vi "TestApplication.vi"() -> ()   [LabVIEW 2016]
uses:
  SEDSpectrometer/FiberSpectrograph.lvclass
  <vilib>/express/express arith-compare/Formula/XNode/ExpressFormulaBlockNode.xnode
panel:
  in  "NrOfAVG":u32=1 caption="Number of averages"
  in  "IntDelay":dbl=-20.0 caption="Integration delay [ns]" min=-20.0 format="%#.0f"
  in  "IntTime":sgl=32.0 caption="Integration time [ms]" format="%.2f"
  out "TecControlType.Setpoint":sgl
  in  "Get Temp Setpoint":bool
  in  "Get Temperature":bool caption="Start Measurement"
  out "Current Temperature":sgl=-6.1035157e-06 format="%_2f"
  in  "Set Parameters":bool caption="Start Measurement"
  in  "Temperature Setpoint":sgl=1.0 format="%_3f"
  out "XY Graph":cluster{"Y":dbl[], "Y":dbl[]}[](graph)
  in  "Exit":bool
  out "Status":string
  in  "StopMeasurement":bool
  in  "StartMeasurement":bool caption="Start Measurement"
  in  "NrOfScans":i16=-1 caption="Nr Of Scans"
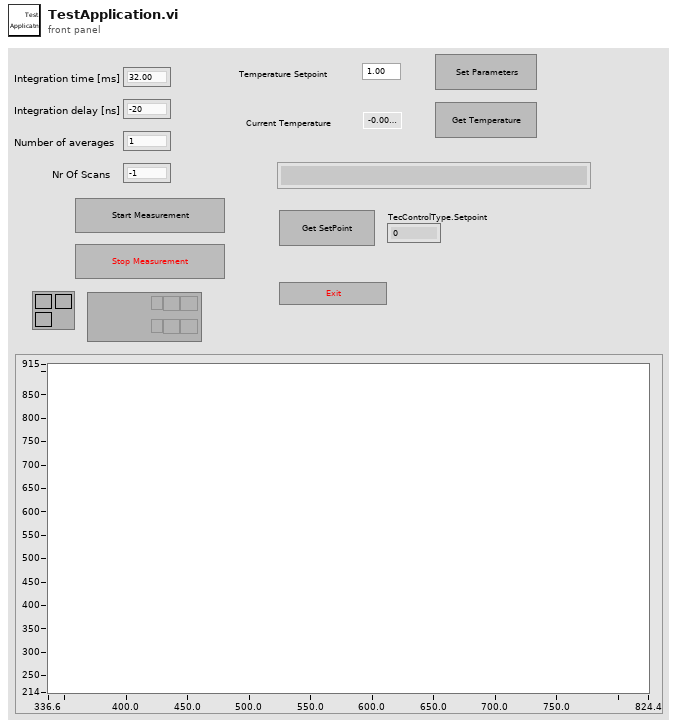
[diagram p1: front panel]
types:
  T1 = cluster{"StartPixel":u16, "StopPixel":u16, "IntegrationTime":sgl, "IntegrationDelay":u32, "NrAverages":u32, "DarkCorrectionType":cluster{"Enable CorDynDark":u8, "ForgetPercentage":u8}, "SmoothingType":cluster{"SmoothPix":u16, "SmoothModel":u8}, "SatDetection":u8, "TriggerType":cluster{"Trigger Mode":u8, "Trigger Source":u8, "Trigger SourceType":u8}, "ControlSettingsType":cluster{"StrobeControl":u16, "LaserDelay":u32, "LaserWidth":u32, "LaserWaveLength":sgl, "StoreToRam":u16}}
  T2 = cluster{"Len":u16, "ConfigVersion":u16, "UserFriendlyId":u8[], "DetectorType":cluster{"SensorType":u8, "NrPixels":u16, "Fit":sgl[], "NLEnable":u8, "NLCorrect":dbl[], "LowNLCounts":dbl, "HighNLCounts":dbl, "Gain":sgl[], "Reserved":sgl, "Offset":sgl[], "Extern Offset":sgl, "DefectivePixels":u16[]}, "IrradianceType":cluster{"SpectrumCalibrationType":cluster{"SmoothingType":cluster{"m_SmoothPix":u16, "SmoothModel":u8}, "CalInttime":sgl, "CalibConvers":sgl[]}, "CalibrationType":u8, "FiberDiameter":i32}, "SpectrumCalibrationType":cluster{"SmoothingType":cluster{"m_SmoothPix":u16, "SmoothModel":u8}, "CalInttime":sgl, "CalibConvers":sgl[]}, "SpectrumCorrectionType":sgl[], "StandAloneType":cluster{"StandAloneType":u8, "MeasConfigType":cluster{"StartPixel":u16, "StopPixel":u16, "IntegrationTime":sgl, "IntegrationDelay":u32, "NrAverages":u32, "DarkCorrectionType":cluster{"Enable CorDynDark":u8, "ForgetPercentage":u8}, "SmoothingType":cluster{"SmoothPix":u16, "SmoothModel":u8}, "SatDetection":u8, "TriggerType":cluster{"Trigger Mode":u8, "Trigger Source":u8, "Trigger SourceType":u8}, "ControlSettingsType":cluster{"StrobeControl":u16, "LaserDelay":u32, "LaserWidth":u32, "LaserWaveLength":sgl, "StoreToRam":u16}}, "Nmsr":i16}, "DynamicStorageType":cluster{"Nmsr":i32, "Reserved":u8[]}, "TempSensorType":sgl[], "TecControlType":cluster{"Enable":u8, "Setpoint":sgl, "Fit[NR_DAC_POL_COEF]":sgl[]}, "ProcessControlType":cluster{"AnalogLow":sgl[], "AnalogHigh":sgl[], "DigitalLow":sgl[], "DigitalHigh":sgl[]}, "EthernetSettingsType":cluster{"IpAddr":u32, "NetMask":u32, "Gateway":u32, "DhcpEnabled":u8, "TcpPort":u16, "LinkStatus":u8}, "Reserved":u8[]}
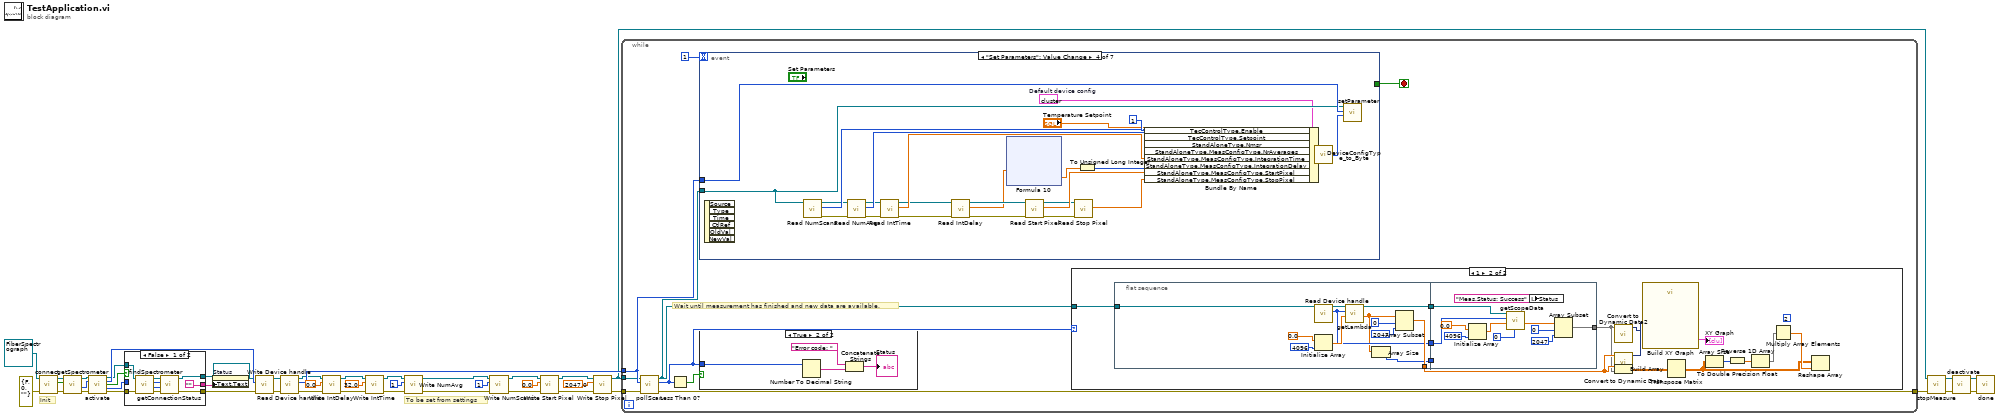
[diagram p0: block diagram]
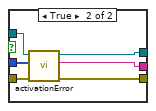
[diagram p2: hidden frame]
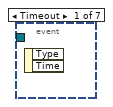
[diagram p5: hidden frame]
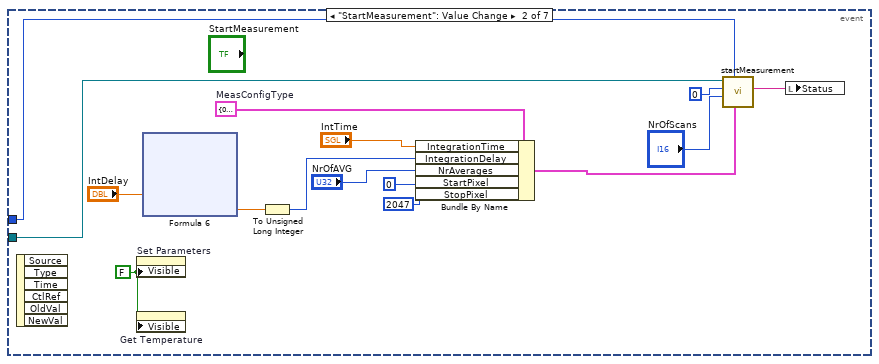
[diagram p6: hidden frame]
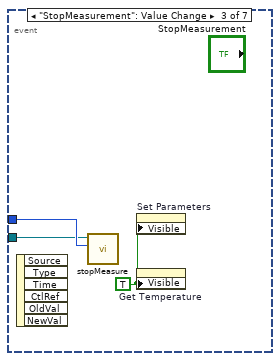
[diagram p7: hidden frame]
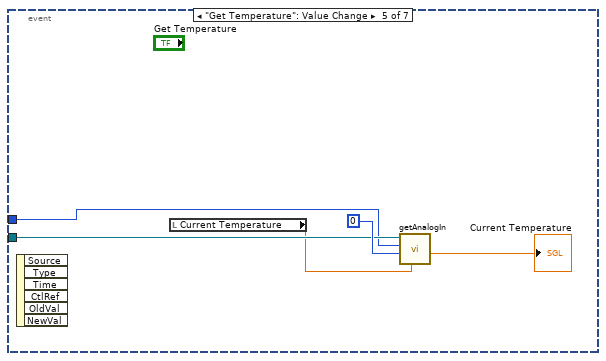
[diagram p8: hidden frame]
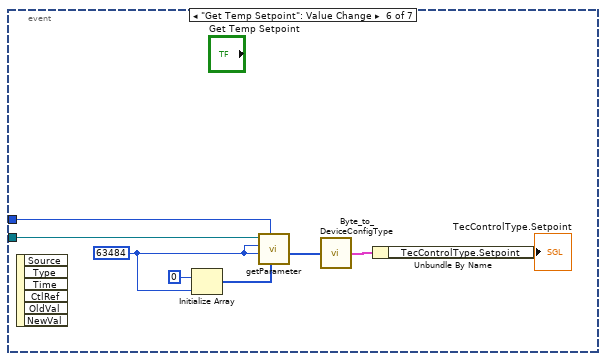
[diagram p9: hidden frame]
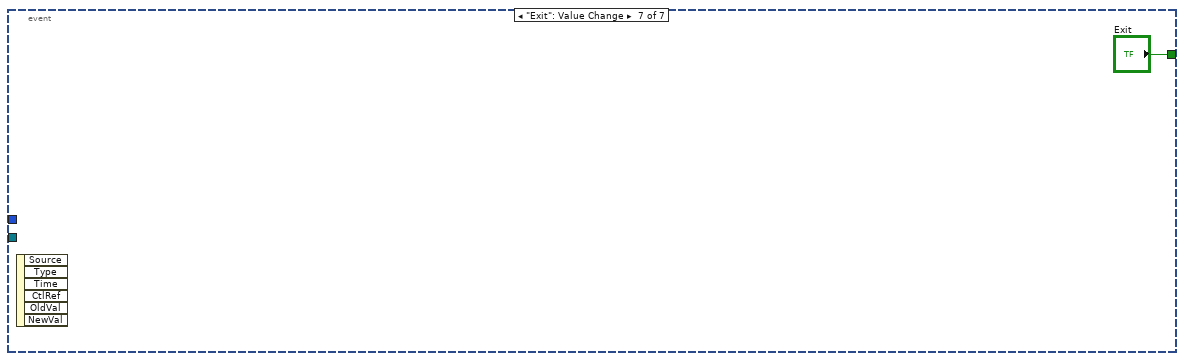
[diagram p10: hidden frame]
diagram:
  # "To be set from settings"
  # "Init"
  n1 = call "connect.vi"("error in (no error)"=errorcluster {"status"=FALSE, "code"=0, "source"=""}, "SEDSpectrometer in"=refnum<class "FiberSpectrograph.lvclass"> refnum) -> ("error out"=w41:errorcluster, "Connected"=w22:bool, "SEDSpectrometer out"=w42:refnum<class "FiberSpectrograph.lvclass">)  [unwired: 7 in]
  n2 = call "getSpectrometer.vi"("error in (no error)"=w41, "Boolean"=w22, "SEDSpectrometer in"=w42) -> ("error out"=w37:errorcluster, "AviableSpec"=w40:u8[], "SEDSpectrometer out"=w36:refnum<class "FiberSpectrograph.lvclass">)  [unwired: 6 in]
  n3 = call "activate.vi"("SEDSpectrometer in"=w36, "DeviceId"=w40, "error in (no error)"=w37) -> ("SEDSpectrometer out"=w30:refnum<class "FiberSpectrograph.lvclass">, "Device handle"=w31:i32, "Activation Error"=w26:bool, "DeviceId"=w27:u8[], "error out"=w29:errorcluster)  [unwired: 8 in]
  n4 = case shown="False" w26 {
    tunnel: w30 -> [w52 w59]
    tunnel: w29 -> [w51 w58]
    tunnel: [w47 w57] -> w24
    tunnel: ["" ("Status") w56] -> w28
    tunnel: w27 -> [_ w55]
    tunnel: [w46 w54] -> w25
    frame False {
      n5 = call "findSpectrometer.vi"("error in (no error)"=w51, "SEDSpectrometer in"=w52) -> ("error out"=w48:errorcluster, "NumOfDevices"=w49:i32, "AviableSpec"=w50:u8[], "SEDSpectrometer out"=w53:refnum<class "FiberSpectrograph.lvclass">)  [unwired: 6 in]
      n6 = call "getConnectionStatus.vi"("SEDSpectrometer in"=w53, "AvailableSpectrometer"=w50, "NumOfDevices"=w49, "error in (no error)"=w48) -> ("SEDSpectrometer out"=w46:refnum<class "FiberSpectrograph.lvclass">, "error out"=w47:errorcluster)  [unwired: 4 in, 1 out]
    }
    frame True {
      n7 = call "activationError.vi"("error in (no error)"=w58, "DeviceId"=w55, "SEDSpectrometer in"=w59) -> ("error out"=w57:errorcluster, "Status"=w56:string, "SEDSpectrometer out"=w54:refnum<class "FiberSpectrograph.lvclass">)  [unwired: 6 in]
    }
  }
  n8 = property on="Status" class="Str"("Text.Text"=w28) -> ()  [unwired: 2 in, 2 out]
  n9 = call-dynamic "Write Device handle.vi"("error in (no error)"=w24, "Device handle"=w31, "SEDSpectrometer in"=w25) -> ("error out"=w35:errorcluster, "SEDSpectrometer out"=w32:refnum<class "FiberSpectrograph.lvclass">)  [unwired: 7 in]
  n10 = call-dynamic "Read Device handle.vi"("error in (no error)"=w35, "SEDSpectrometer in"=w32) -> ("error out"=w7:errorcluster, "Device handle"=w21:i32, "SEDSpectrometer out"=w2:refnum<class "FiberSpectrograph.lvclass">)  [unwired: 7 in]
  n11 = call-dynamic "Write IntDelay.vi"("error in (no error)"=w7, "IntDelay"=0.0, "SEDSpectrometer in"=w2) -> ("error out"=w15:errorcluster, "SEDSpectrometer out"=w20:refnum<class "FiberSpectrograph.lvclass">)  [unwired: 7 in]
  n12 = call-dynamic "Write IntTime.vi"("error in (no error)"=w15, "IntTime"=sgl 32.0, "SEDSpectrometer in"=w20) -> ("error out"=w14:errorcluster, "SEDSpectrometer out"=w19:refnum<class "FiberSpectrograph.lvclass">)  [unwired: 7 in]
  n13 = call-dynamic "Write NumAvg.vi"("error in (no error)"=w14, "NumAvg"=u32 1, "SEDSpectrometer in"=w19) -> ("error out"=w13:errorcluster, "SEDSpectrometer out"=w18:refnum<class "FiberSpectrograph.lvclass">)  [unwired: 7 in]
  n14 = call-dynamic "Write NumScans.vi"("error in (no error)"=w13, "NumScans"=i16 1, "SEDSpectrometer in"=w18) -> ("error out"=w12:errorcluster, "SEDSpectrometer out"=w17:refnum<class "FiberSpectrograph.lvclass">)  [unwired: 7 in]
  n15 = call-dynamic "Write Start Pixel.vi"("error in (no error)"=w12, "Start Pixel"=0.0, "SEDSpectrometer in"=w17) -> ("error out"=w11:errorcluster, "SEDSpectrometer out"=w16:refnum<class "FiberSpectrograph.lvclass">)  [unwired: 7 in]
  n16 = call-dynamic "Write Stop Pixel .vi"("error in (no error)"=w11, "Stop Pixel"=2047.0, "SEDSpectrometer in"=w16) -> ("error out"=w6:errorcluster, "SEDSpectrometer out"=w1:refnum<class "FiberSpectrograph.lvclass">)  [unwired: 7 in]
  n17 = while {
    tunnel: w21 -> [w61]
    tunnel: w6 -> [w65]
    tunnel: [w64] -> w23
    tunnel: w1 -> [w60]
    stop <- w66 stop-if-true
    # "Wait until measurement has finished and new data are available."
    n18 = call "pollScan.vi"("error in (no error)"=w65, "Device"=w61, "SEDSpectrometer in"=w60) -> ("error out"=w64:errorcluster, "Output Value"=w62:i32, "SEDSpectrometer out"=w63:refnum<class "FiberSpectrograph.lvclass">)  [unwired: 6 in]
    n19 = Less Than 0?(x=w62) -> (x < 0?=w67:bool)
    n20 = event shown="[3] \"Set Parameters\": Value Change" {
      selector: _ -> [_ _ _ _ _ _ _]
      dyn-events: _ -> [_ _ _ _ _ _ _]
      timeout: 1 -> [_ _ _ _ _ _ _]
      tunnel: [_ _ _ _ _ _ "Exit"] -> w66
      tunnel: w61 -> [_ w125 w136 w144 w172 w178 _]
      tunnel: w63 -> [_ w121 w135 w143 w173 w175 _]
      event Timeout {
        n21 = event-data() -> ()  [unwired: 1 in, 2 out]
      }
      event "StartMeasurement": Value Change {
        w119 = T1 {"StartPixel"=0, "StopPixel"=0, "IntegrationTime"=0.0, "IntegrationDelay"=0, "NrAverages"=0, "DarkCorrectionType"={"Enable CorDynDark"=0, "ForgetPercentage"=0}, "SmoothingType"={"SmoothPix"=0, "SmoothModel"=0}, "SatDetection"=0, "TriggerType"={"Trigger Mode"=0, "Trigger Source"=0, "Trigger SourceType"=0}, "ControlSettingsType"={"StrobeControl"=0, "LaserDelay"=0, "LaserWidth"=0, "LaserWaveLength"=0.0, "StoreToRam"=0}}  # MeasConfigType
        w120 = FALSE ("Visible")
        n22 = event-data() -> ()  [unwired: 1 in, 6 out]
        n23 = property on="Set Parameters" class="Bool"("Visible"=w120) -> ()  [unwired: 2 in, 2 out]
        n24 = property on="Get Temperature" class="Bool"("Visible"=w120) -> ()  [unwired: 2 in, 2 out]
        n25 = xnode "Formula 6"("X1"="IntDelay") -> ("Result"=w116:dbl)  [unwired: 1 in, 1 out]
        n26 = To Unsigned Long Integer(number=w116) -> (unsigned 32bit integer=w115:u32)
        n27 = Bundle By Name(cluster=w119, "IntegrationTime"="IntTime", "IntegrationDelay"=w115, "NrAverages"="NrOfAVG", "StartPixel"=u16 0, "StopPixel"=2047 ("length")) -> (w111:T1)
        n28 = call "startMeasurement.vi"("MeasConfigType"=w111, "Device Handle"=w125, "NumOfScans"="NrOfScans", "a_hWnd"=0, "SEDSpectrometer in"=w121) -> ("Status"=w122:string)  [unwired: 3 in, 3 out]
        n29 = local write "Status"(w122) -> ()
      }
      event "StopMeasurement": Value Change {
        w134 = TRUE ("Visible")
        n30 = event-data() -> ()  [unwired: 1 in, 6 out]
        n31 = call "stopMeasure.vi"("Device"=w136, "SEDSpectrometer in"=w135) -> ()  [unwired: 7 in, 3 out]
        n32 = property on="Set Parameters" class="Bool"("Visible"=w134) -> ()  [unwired: 2 in, 2 out]
        n33 = property on="Get Temperature" class="Bool"("Visible"=w134) -> ()  [unwired: 2 in, 2 out]
      }
      event "Set Parameters": Value Change {
        w140 = T2 {"Len"=63484, "ConfigVersion"=3, "UserFriendlyId"=[49, 54, 48, 54, 49, 57, 50, 85, 49, 0, 48, 0, 28, 0, 0, 0, 42, 2, 0, 0, 160, 188, 0, 0, 0, 28, 0, 6, 132, 159, 116, 3, 172, 0, 116, 6, 140, 0, 0, 0, 0, 0, 0, 255, 8, 0, 67, 176, 96, 0, 252, 0, 0, 0, 254, 175, 38, 0, 0, 0, 184, 239, 0, 0], "DetectorType"={"SensorType"=11, "NrPixels"=2048, "Fit"=[314.9799, 0.2943957, -9.917037e-06, -1.0080056e-09, 0.0], "NLEnable"=0, "NLCorrect"=[0.0, 0.0, 0.0, 0.0, 0.0, 0.0, 0.0, 0.0], "LowNLCounts"=0.0, "HighNLCounts"=0.0, "Gain"=[1.277, 1.0], "Reserved"=0.0, "Offset"=[-0.01, 0.0], "Extern Offset"=0.0, "DefectivePixels"=[4095, 4095, 4095, 4095, 4095, 4095, 4095, 4095, 4095, 4095, 4095, 4095, 4095, 4095, 4095, 4095, 4095, 4095, 4095, 4095, 4095, 4095, 4095, 4095, 4095, 4095, 4095, 4095, 4095, 4095]}, "IrradianceType"={"SpectrumCalibrationType"={"SmoothingType"={"m_SmoothPix"=0, "SmoothModel"=0}, "CalInttime"=0.0, "CalibConvers"=array[4096 elements]}, "CalibrationType"=0, "FiberDiameter"=0}, "SpectrumCalibrationType"={"SmoothingType"={"m_SmoothPix"=0, "SmoothModel"=0}, "CalInttime"=0.0, "CalibConvers"=array[4096 elements]}, "SpectrumCorrectionType"=array[4096 elements], "StandAloneType"={"StandAloneType"=0, "MeasConfigType"={"StartPixel"=0, "StopPixel"=2047, "IntegrationTime"=32.0, "IntegrationDelay"=0, "NrAverages"=1, "DarkCorrectionType"={"Enable CorDynDark"=1, "ForgetPercentage"=100}, "SmoothingType"={"SmoothPix"=0, "SmoothModel"=0}, "SatDetection"=1, "TriggerType"={"Trigger Mode"=0, "Trigger Source"=0, "Trigger SourceType"=0}, "ControlSettingsType"={"StrobeControl"=0, "LaserDelay"=0, "LaserWidth"=0, "LaserWaveLength"=0.0, "StoreToRam"=0}}, "Nmsr"=-1}, "DynamicStorageType"={"Nmsr"=0, "Reserved"=[0, 0, 0, 0, 0, 0, 0, 0]}, "TempSensorType"=[118.68976, -70.361015, 21.019672, -3.6442714, 0.1992981, 0.0, 0.0, 0.0, 0.0, 0.0, 51.4, -16.38, 0.0, 0.0, 0.0], "TecControlType"={"Enable"=1, "Setpoint"=1.0, "Fit[NR_DAC_POL_COEF]"=[0.0, 0.0]}, "ProcessControlType"={"AnalogLow"=[0.0, 0.0], "AnalogHigh"=[0.0, 0.0], "DigitalLow"=[0.0, 0.0, 0.0, 0.0, 0.0, 0.0, 0.0, 0.0, 0.0, 0.0], "DigitalHigh"=[0.0, 0.0, 0.0, 0.0, 0.0, 0.0, 0.0, 0.0, 0.0, 0.0]}, "EthernetSettingsType"={"IpAddr"=0, "NetMask"=0, "Gateway"=0, "DhcpEnabled"=0, "TcpPort"=0, "LinkStatus"=0}, "Reserved"=array[13815 elements]}  # Default device config
        n34 = event-data() -> ()  [unwired: 1 in, 6 out]
        n35 = call-dynamic "Read NumScans.vi"("SEDSpectrometer in"=w143) -> ("error out"=w158:errorcluster, "NumScans"=w159:i16, "SEDSpectrometer out"=w157:refnum<class "FiberSpectrograph.lvclass">)  [unwired: 8 in]
        n36 = call-dynamic "Read NumAvg.vi"("error in (no error)"=w158, "SEDSpectrometer in"=w157) -> ("error out"=w155:errorcluster, "NumAvg"=w156:u32, "SEDSpectrometer out"=w154:refnum<class "FiberSpectrograph.lvclass">)  [unwired: 7 in]
        n37 = call-dynamic "Read IntTime.vi"("error in (no error)"=w155, "SEDSpectrometer in"=w154) -> ("error out"=w152:errorcluster, "IntTime"=w153:sgl, "SEDSpectrometer out"=w151:refnum<class "FiberSpectrograph.lvclass">)  [unwired: 7 in]
        n38 = call-dynamic "Read IntDelay.vi"("error in (no error)"=w152, "SEDSpectrometer in"=w151) -> ("error out"=w150:errorcluster, "IntDelay"=w138:dbl, "SEDSpectrometer out"=w149:refnum<class "FiberSpectrograph.lvclass">)  [unwired: 7 in]
        n39 = xnode "Formula 10"("X1"=w138) -> ("Result"=w139:dbl)  [unwired: 1 in, 1 out]
        n40 = call-dynamic "Read Start Pixel.vi"("error in (no error)"=w150, "SEDSpectrometer in"=w149) -> ("error out"=w147:errorcluster, "Start Pixel"=w148:dbl, "SEDSpectrometer out"=w146:refnum<class "FiberSpectrograph.lvclass">)  [unwired: 7 in]
        n41 = call-dynamic "Read Stop Pixel .vi"("error in (no error)"=w147, "SEDSpectrometer in"=w146) -> ("Stop Pixel"=w145:dbl)  [unwired: 7 in, 2 out]
        n42 = To Unsigned Long Integer(number=w139) -> (unsigned 32bit integer=w137:u32)
        n43 = Bundle By Name(cluster=w140, "TecControlType.Enable"=u8 1, "TecControlType.Setpoint"="Temperature Setpoint", "StandAloneType.Nmsr"=w159, "StandAloneType.MeasConfigType.NrAverages"=w156, "StandAloneType.MeasConfigType.IntegrationTime"=w153, "StandAloneType.MeasConfigType.IntegrationDelay"=w137, "StandAloneType.MeasConfigType.StartPixel"=w148, "StandAloneType.MeasConfigType.StopPixel"=w145) -> (w142:T2)
        n44 = call "DeviceConfigType_to_Byte.vi"("DeviceConfig"=w142) -> ("Byte Array"=w141:u8[])  [unwired: 4 in]
        n45 = call "setParameter.vi"("DeviceParm"=w141, "Device"=w144, "SEDSpectrometer in"=w143) -> ()  [unwired: 5 in, 4 out]
      }
      event "Get Temperature": Value Change {
        n46 = event-data() -> ()  [unwired: 1 in, 6 out]
        n47 = local read "Current Temperature"() -> (w170:sgl)
        n48 = call "getAnalogIn.vi"("AnalogIn"=w170, "AnalogInId"=0 ("Device"), "Device"=w172, "SEDSpectrometer in"=w173) -> ("AnalogIn"=→"Current Temperature":sgl)  [unwired: 4 in, 3 out]
      }
      event "Get Temp Setpoint": Value Change {
        w181 = u16 63484 ("a_pNumPixelsInput")
        n49 = event-data() -> ()  [unwired: 1 in, 6 out]
        n50 = Initialize Array(u8 0, w181) -> (w180:u8[])
        n51 = call "getParameter.vi"("DeviceParm"=w180, "Device handle"=w178, "RequiredSizeInput"=w181, "Size"=w181, "SEDSpectrometer in"=w175) -> ("DeviceParam"=w179:u8[])  [unwired: 2 in, 4 out]
        n52 = call "Byte_to_DeviceConfigType.vi"("Byte Array"=w179) -> ("output cluster"=w177:T2)  [unwired: 4 in]
        n53 = Unbundle By Name(w177) -> ("TecControlType.Setpoint"=→"TecControlType.Setpoint":sgl)
      }
      event "Exit": Value Change {
        n54 = event-data() -> ()  [unwired: 1 in, 6 out]
      }
    }
    n55 = case shown="True" w67 {
      tunnel: w62 -> [_ w108]
      frame False {
      }
      frame True {
        n56 = Number To Decimal String(number=w108) -> (decimal integer string=w109:string)  [unwired: 1 in]
        n57 = Concatenate Strings("Error code: ", w109) -> (→"Status":string)
      }
    }
    n58 = case shown="1" w62 {
      tunnel: w63 -> [_ w80]
      frame 0, Default {
      }
      frame 1 {
        (unwired) 2 ("naxis")
        n59 = flat-sequence {
          tunnel: w80 -> [w89]
          tunnel: [w90] -> w76
          tunnel: [w88] -> w79
          tunnel: [w86] -> w78
          tunnel: [w84] -> w77
          tunnel: [w100] -> w75
          tunnel: w79 -> [w98]
          tunnel: w78 -> [w97]
          tunnel: w77 -> [_]
          frame #0 {
            n60 = call-dynamic "Read Device handle.vi"("SEDSpectrometer in"=w89) -> ("Device handle"=w88:i32, "SEDSpectrometer out"=w87:refnum<class "FiberSpectrograph.lvclass">)  [unwired: 8 in, 1 out]
            n61 = Initialize Array(0.0, 4096 ("dimension size")) -> (w93:dbl[])
            n62 = call "getLambda.vi"("WaveLength In"=w93, "Device"=w88, "SEDSpectrometer in"=w87) -> ("WaveLength Out"=w85:dbl[], "SEDSpectrometer out"=w86:refnum<class "FiberSpectrograph.lvclass">)  [unwired: 5 in, 2 out]
            n63 = Array Size(array=w85) -> (size(s)=w84:i32)
            n64 = Array Subset(array=w85, index=0, length=2047) -> (w90:dbl[])
          }
          frame #1 {
            n65 = Initialize Array(0.0 ("element"), 4096 ("dimension size")) -> (w102:dbl[])
            n66 = call "getScopeData.vi"("TimeLabel"=u32 0, "Spectrum"=w102, "Device"=w98, "SEDSpectrometer in"=w97) -> ("Spectrum"=w96:dbl[])  [unwired: 4 in, 3 out]
            n67 = local write "Status"("Meas.Status: Success" ("Status")) -> ()
            n68 = Array Subset(array=w96, index=0, length=2047) -> (w100:dbl[])
          }
        }
        n69 = call "Convert to Dynamic Data2"("Array"=w75) -> ("Dynamic Data Type"=w82:dynamicdata)  [unwired: 3 in]
        n70 = call "Convert to Dynamic Data"("Array"=w76) -> ("Dynamic Data Type"=w83:dynamicdata)  [unwired: 3 in]
        n71 = Build Array(w76, w75) -> (w71:dbl[][])
        n72 = call "Build XY Graph"("Y Input"=w82, "X Input"=w83) -> ("XY Graph"=→"XY Graph":cluster{"Y":dbl[], "Y":dbl[]}[])  [unwired: 8 in, 1 out]
        n73 = Transpose Matrix(1:w71) -> (0:w69:dbl[][])
        n74 = Array Size(array=w69) -> (size(s)=w73:i32[])
        n75 = To Double Precision Float(number=w73) -> (double precision float=w70:dbl[])
        n76 = Reverse 1D Array(array=w70) -> (reversed array=w72:dbl[])
        n77 = Multiply Array Elements(1:w72) -> (0:w74:dbl)
        n78 = Reshape Array(w69, w74) -> ()  [unwired: 1 out]
      }
    }
  }
  n79 = call "stopMeasure.vi"("error in (no error)"=w23, "SEDSpectrometer in"=w1) -> ("error out"=w33:errorcluster, "SEDSpectrometer out"=w34:refnum<class "FiberSpectrograph.lvclass">)  [unwired: 7 in, 1 out]
  n80 = call "deactivate.vi"("error in (no error)"=w33, "SEDSpectrometer in"=w34) -> ("error out"=w39:errorcluster, "SEDSpectrometer out"=w38:refnum<class "FiberSpectrograph.lvclass">)  [unwired: 7 in, 1 out]
  n81 = call "done.vi"("error in (no error)"=w39, "SEDSpectrometer in"=w38) -> ()  [unwired: 7 in, 3 out]
